vi "Test MQTT-6.0.0-1.vi"(8 "error in (no error)":errorcluster, 11 "Connection Config":refnum<class "Connection.lvclass">) -> (0 "error out":errorcluster, 3 "Connection Config dup":refnum<class "Connection.lvclass">)   [LabVIEW 2013]
uses:
  <vilib>/LabVIEW Open Source Project/MQTT Connection/MQTT_Connection/Connection/Connection.lvclass
  <vilib>/LabVIEW Open Source Project/MQTT Control Packets/Control Packets/ControlPacket/Control Packet Type -- enum.ctl
  <vilib>/LabVIEW Open Source Project/MQTT Control Packets/Control Packets/ControlPacket/QualityOfService -- enum.ctl
  <vilib>/LabVIEW Open Source Project/MQTT Websockets Connection/MQTT_Websockets/Connection/WebsocketsConnection.lvclass
  <vilib>/addons/_JKI Toolkits/Caraya/classes/Test/Test.lvclass
  <vilib>/LabVIEW Open Source Project/MQTT Control Packets/Control Packets/CONNECT/CONNECT.lvclass
  <vilib>/LabVIEW Open Source Project/MQTT Control Packets/Control Packets/PUBLISH/PUBLISH.lvclass
  <vilib>/LabVIEW Open Source Project/MQTT Control Packets/Control Packets/ControlPacket/ControlPacket.lvclass
  <vilib>/addons/_JKI Toolkits/Caraya/classes/Assert/Assert.lvclass
panel:
  out "Should not receive Puback":T1
  out "Connack Packet received?":T1
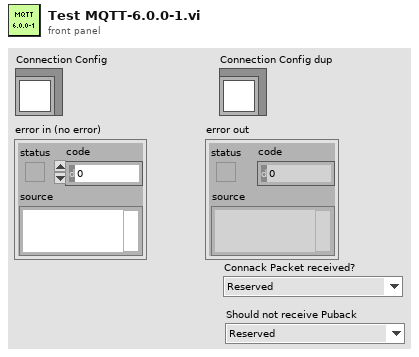
[diagram p1: front panel]
types:
  T1 = typedef "MQTT_Control_Packets.lvlib/ControlPacket.lvclass/Control Packet Type -- enum.ctl" = enum16{"Reserved", "CONNECT", "CONNACK", "PUBLISH", "PUBACK", "PUBREC", "PUBREL", "PUBCOMP", "SUBSCRIBE", "SUBACK", "UNSUBSCRIBE", "UNSUBACK", "PINGREQ", "PINGRESP", "DISCONNECT", "AUTH"}
  T2 = typedef "MQTT_Control_Packets.lvlib/ControlPacket.lvclass/QualityOfService -- enum.ctl" = enum16{"0 (At Most Once)", "1 (At Least Once)", "2 (Exactly Once)"}
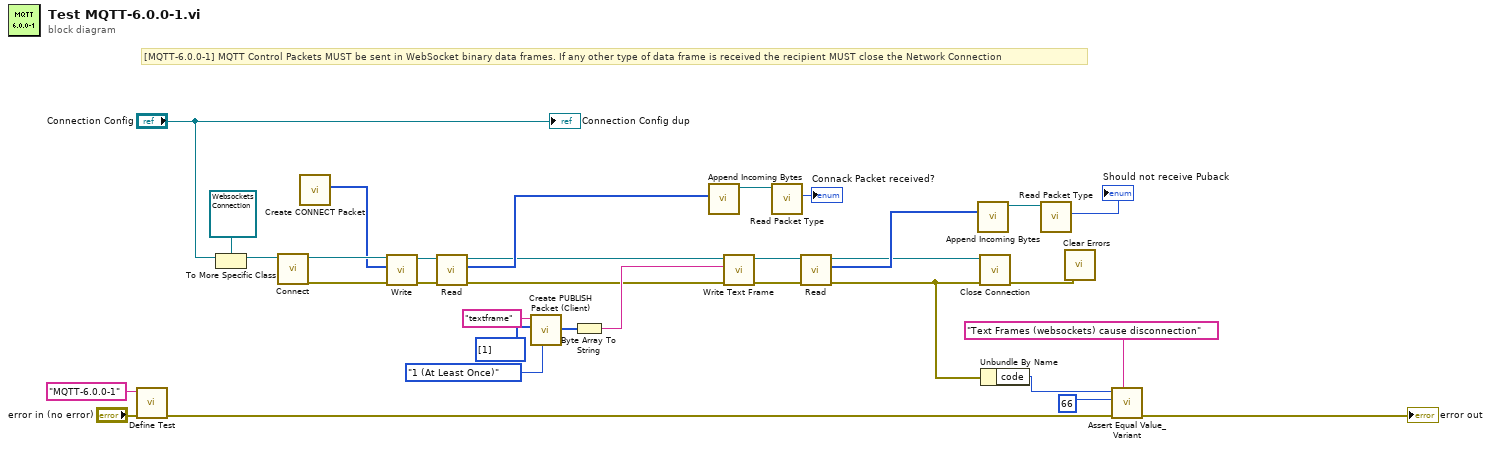
[diagram p0: block diagram]
diagram:
  # "[MQTT-6.0.0-1] MQTT Control Packets MUST be sent in WebSocket binary data frames. If any other type of data frame is received the recipient MUST close the Network Connection"
  n1 = call <vilib>:"Define Test.vi"("error in (no error)"="error in (no error)", "Label (VI Title)"="MQTT-6.0.0-1") -> ("error out"=w28:errorcluster)  [unwired: 9 in]
  n2 = To More Specific Class(target class=refnum<class "WebsocketsConnection.lvclass"> refnum ("WebsocketsConnection in"), reference="Connection Config") -> (specific class reference=w10:refnum<class "WebsocketsConnection.lvclass">)  [unwired: 1 in, 1 out]
  n3 = call <vilib>:"Connect.vi"("Connection in"=w10) -> ("error out"=w15:errorcluster, "Connection out"=w17:refnum<class "WebsocketsConnection.lvclass">)  [unwired: 9 in]
  n4 = call <vilib>:"Create CONNECT Packet.vi"() -> ("Bytes Stream"=w16:u8[])  [unwired: 9 in, 2 out]
  n5 = call <vilib>:"Write.vi"("error in (no error)"=w15, "Bytes"=w16, "Connection in"=w17) -> ("error out"=w14:errorcluster, "Connection"=w13:refnum<class "WebsocketsConnection.lvclass">)  [unwired: 7 in]
  n6 = call <vilib>:"Read.vi"("error in (no error)"=w14, "TCPConnection in"=w13) -> ("error out"=w5:errorcluster, "Bytes"=w12:u8[], "TCPConnection out"=w11:refnum<class "WebsocketsConnection.lvclass">)  [unwired: 5 in, 2 out]
  n7 = call <vilib>:"Create PUBLISH Packet (Client).vi"("QoS"=QualityOfService_--_enum."1 (At Least Once)", "Payload"=u8[] [1], "Topic Name"="textframe") -> ("Bytes Stream"=w26:u8[])  [unwired: 5 in, 3 out]
  n8 = Byte Array To String(unsigned byte array=w26) -> (string=w8:string)
  n9 = call <vilib>:"Append Incoming Bytes.vi"("Incoming Packets"=w12) -> ("ControlPacket"=w25:refnum<class "ControlPacket.lvclass">)  [unwired: 7 in, 3 out]
  n10 = call <vilib>:"Write Text Frame.vi"("error in (no error)"=w5, "Text"=w8, "WebsocketsConnection in"=w11) -> ("error out"=w4:errorcluster, "WebsocketsConnection out"=w7:refnum<class "WebsocketsConnection.lvclass">)  [unwired: 7 in]
  n11 = call <vilib>:"Read Packet Type.vi"("ControlPacket in"=w25) -> ("Control Packet Type"=→"Connack Packet received?":T1)  [unwired: 9 in, 1 out]
  n12 = call <vilib>:"Read.vi"("error in (no error)"=w4, "TCPConnection in"=w7) -> ("error out"=w2:errorcluster, "Bytes"=w6:u8[], "TCPConnection out"=w3:refnum<class "WebsocketsConnection.lvclass">)  [unwired: 5 in, 2 out]
  n13 = call <vilib>:"Append Incoming Bytes.vi"("Incoming Packets"=w6) -> ("ControlPacket"=w23:refnum<class "ControlPacket.lvclass">)  [unwired: 7 in, 3 out]
  n14 = call <vilib>:"Close Connection.vi"("error in (no error)"=w2, "Connection in"=w3) -> ("error out"=w1:errorcluster)  [unwired: 8 in, 1 out]
  n15 = Unbundle By Name(w2) -> ("code"=w21:i32)
  n16 = call <vilib>:"Read Packet Type.vi"("ControlPacket in"=w23) -> ("Control Packet Type"=→"Should not receive Puback":T1)  [unwired: 9 in, 1 out]
  n17 = call <vilib>:"Clear Errors.vi"("error in (no error)"=w1) -> ()  [unwired: 6 in, 1 out]
  n18 = call <vilib>:"Assert Equal Value_Variant.vi"("Label"="Text Frames (websockets) cause disconnection", "error in (no error)"=w28, "Y"=66 ("code"), "X"=w21) -> ("error out"=→"error out":errorcluster)  [unwired: 7 in]
  "Connection Config dup" <- "Connection Config"
